vi "CTRE_Phoenix_Pigeon2_ClearStickyFaults.vi"(6 "timeoutMs":i32, 8 "error in":errorcluster, 11 "PigeonIMUDevRef 2":T1={"DeviceStatus"={"status"=FALSE, "code"=0, "source"=""}, "Device Number"=0, "Type"=352321536, "Device ID"=0, "Handle"=0, "UsageFrame"=0, "Library Path"=path ""} {"Type" items=["CAN"=352321536, "TalonSRX"=33554432]}) -> (0 "error out":errorcluster, 3 "PigeonIMUDevRef":T1={"DeviceStatus"={"status"=FALSE, "code"=0, "source"=""}, "Device Number"=0, "Type"=352321536, "Device ID"=0, "Handle"=0, "UsageFrame"=0, "Library Path"=path ""} {"Type" items=["CAN"=352321536, "TalonSRX"=33554432]})   [LabVIEW 2020]
doc: "Clears the sticky faults from a Pigeon2."
uses:
  <vilib>/Rock Robotics/WPI/ThirdParty/Phoenix-LabVIEW/Pigeon IMU/CTRE_PigeonIMU_ConnectionType.ctl
  <vilib>/Rock Robotics/WPI/ThirdParty/Phoenix-LabVIEW/Pigeon IMU/CTRE_PigeonIMU_DeviceRef.ctl
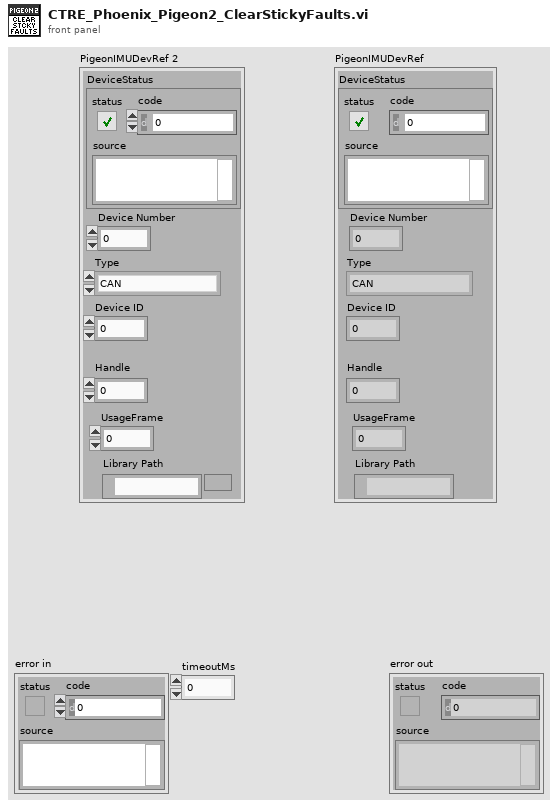
[diagram p1: front panel]
types:
  T1 = typedef "CTRE_PigeonIMU_DeviceRef.ctl" = cluster{"DeviceStatus":errorcluster, "Device Number":u8, "Type":T2, "Device ID":u32, "Handle":u64, "UsageFrame":u32, "Library Path":path}
  T2 = typedef "CTRE_PigeonIMU_ConnectionType.ctl" = u32
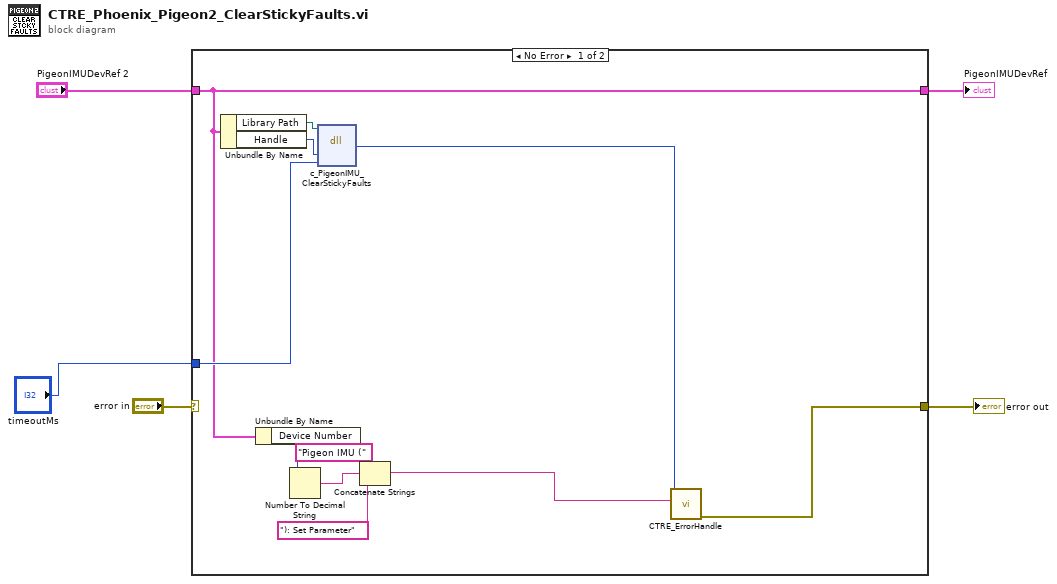
[diagram p0: block diagram]
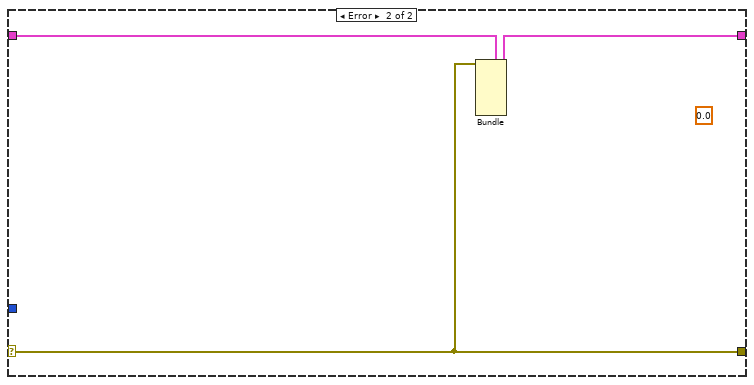
[diagram p2: hidden frame]
diagram:
  n1 = case shown="No Error" "error in" {
    selector: "error in" -> [_ w18]
    tunnel: "PigeonIMUDevRef 2" -> [w8 w19]
    tunnel: [w16 w18] -> w5
    tunnel: [w8 w17] -> w1
    tunnel: "timeoutMs" -> [w9 _]
    frame No Error {
      n2 = Unbundle By Name(w8) -> ("Library Path"=w7:path, "Handle"=w6:u64)
      n3 = Unbundle By Name(w8) -> ("Device Number"=w12:u8)
      n4 = Number To Decimal String(number=w12) -> (decimal integer string=w14:string)  [unwired: 1 in]
      n5 = dll-call lib="?" fn="c_PigeonIMU_ClearStickyFaults"(path in=w7, "handle"=w6, "timeoutMs"=w9) -> ("return type"=w11:i32)  [unwired: 4 in, 2 out]
      n6 = Concatenate Strings("Pigeon IMU (" ("string"), w14, "): Set Parameter" ("string")) -> (w10:string)
      n7 = call <vilib>:"CTRE_ErrorHandle.vi"("origin"=w10, "code"=w11) -> ("error out"=w16:errorcluster)  [unwired: 9 in]
    }
    frame Error {
      (unwired) sgl 0.0 ("value")
      n8 = Bundle(cluster=w19, "DeviceStatus"=w18) -> (w17:T1)  [unwired: 6 in]
    }
  }
  "error out" <- w5
  "PigeonIMUDevRef" <- w1
